vi "AUTOFOCUS_save_new_PID_parameters.vi"(2 "error in":errorcluster, 3 "Autofocus cluster":T1, 4 "PID gains":T2, 5 "queue MAIN":refnum<queue>) -> (0 "error out":errorcluster, 1 "Autofocus cluster OUT":T1)   [LabVIEW 2015]
uses:
  CONTROLS/Q_main_element.ctl
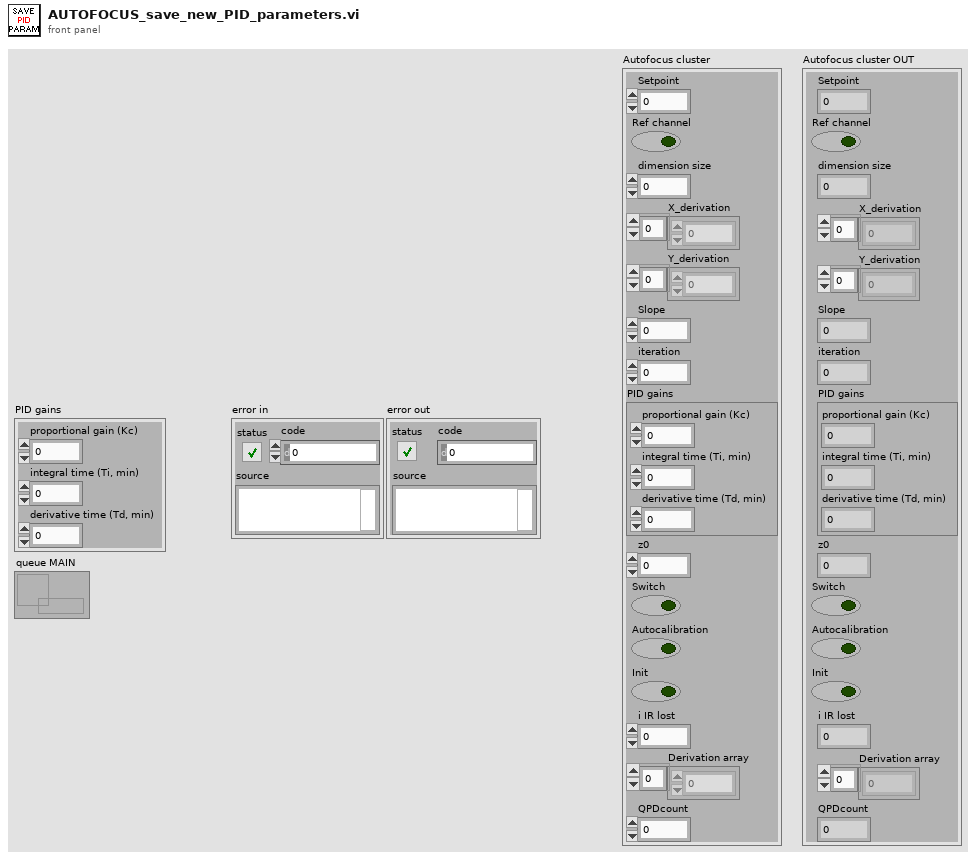
[diagram p1: front panel]
types:
  T1 = cluster{"Setpoint":dbl, "Ref channel":bool, "dimension size":i32, "X_derivation":dbl[], "Y_derivation":dbl[], "Slope":dbl, "iteration":i32, "PID gains":cluster{"proportional gain (Kc)":dbl, "integral time (Ti, min)":dbl, "derivative time (Td, min)":dbl}, "z0":dbl, "Switch":bool, "Autocalibration":bool, "Init":bool, "i IR lost":i32, "Derivation array":dbl[], "QPDcount":u32}
  T2 = cluster{"proportional gain (Kc)":dbl, "integral time (Ti, min)":dbl, "derivative time (Td, min)":dbl}
  T3 = typedef "Q_main_element.ctl" = cluster{"variant":variant, "Instruction":enum16{"Main_idle", "Main_initialize", "Main_initialize_TDMS", "Main_initialize_Queue", "Main_error", "Main_DAQ_initialization_results", "Main_ASI_initialization_results", "Main_Piezo_initialization_results", "Main_Valve_initialization_results", "Main_Pump_initialization_results", "Main_CAMERA_initialization_results", "Main_FPGA_initialization_results", "Main_DAQ_error", "Main_ASI_error", "Main_Piezo_error", "Main_CAMERA_error", "Main_Valve_error", "Main_Pump_error", "Main_FPGA_error", "Main_start_acquiring", "Main_not_acquiring", "Main_acquiring", "Main_stop_acquiring", "Main_change_exposure", "Main_change_z_scan_parameters", "Main_define_ROI", "Main_define_mosaic", "Main_read_kinetic_time", "Main_cooler", "Main_read_temperature", "Main_save_XY", "Main_load_XY", "Main_discard_XY", "Main_move_to_XY", "Main_measure_QPD", "Main_autofocus_calibration", "Main_autofocus_initialization", "Main_autofocus_stop", "Main_save_PID", "Main_change_H_valve_position", "Main_two_way_valve", "Main_save_movie", "Main_init_single_scan", "Main_single_scan", "Main_stop_single_scan", "Main_merFISH_illumination_parameters", "Main_merFISH_buffer_probe_list", "Main_merFISH_injections_procedure", "Main_merFISH_save_setpoint", "Main_merFISH_DAPI_parameters", "Main_merFISH_Brightfield_parameters", "Main_merFISH_save_embryo_ROI", "Main_merFISH_init", "Main_merFISH_resume", "Main_merFISH_start_autofocus", "Main_merFISH_open_close_valve_merFISH", "Main_merFISH_open_close_valve_photobleaching", "Main_merFISH_hybridization", "Main_merFISH_move_to_ROI", "Main_merFISH_wait_stabilization", "Main_merFISH_move_to_REF", "Main_merFISH_scan", "Main_merFISH_photobleaching_injection", "Main_merFISH_photobleaching", "Main_merFISH_send_email", "Main_merFISH_close", "Main_STOP"}}
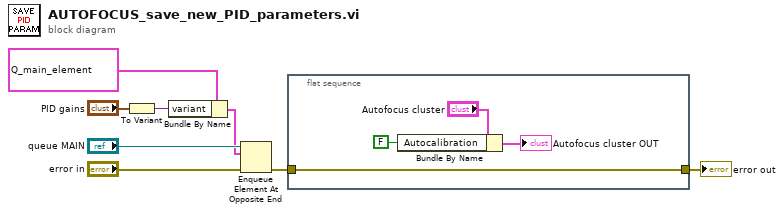
[diagram p0: block diagram]
diagram:
  n1 = To Variant(anything="PID gains") -> (Variant=w5:variant)
  n2 = Bundle By Name(cluster=T3 {"variant"=variant, "Instruction"=enum."Main_save_PID"} ("Q_main_element"), "variant"=w5) -> (w3:T3)
  n3 = Enqueue Element At Opposite End(queue="queue MAIN", element=w3, error in (no error)="error in") -> (error out=w2:errorcluster)  [unwired: 1 in, 2 out]
  n4 = flat-sequence {
    tunnel: w2 -> [w10]
    tunnel: [w10] -> w1
    frame #0 {
      n5 = Bundle By Name(cluster="Autofocus cluster", "Autocalibration"=FALSE) -> ()  [unwired: 1 out]
      "Autofocus cluster OUT" <- "Autofocus cluster"
    }
  }
  "error out" <- w1
